vi "Initiate and Generate (Multi).vi"(0 "niUsrpRio Sessions":T3[](array[typedef]) {"FPGA Data Clock Rate" format="%#.3pHz"; "Data Clock Rate" format="%#.3pHz"; "Characterization Data"."Frequencies [Hz]" format="%#_6p"; "EEPROM Characterization Header"."Pointer to Device Data Header" format="%x"; "EEPROM Characterization Header"."Checksum" format="%x"; "Device Data Header"."Pointer to Characterization Data" format="%x"; "Device Data Header"."Checksum" format="%x"; "EEPROM Header"."Pointer to User Header" format="%x"; "EEPROM Header"."Pointer to Factory Header" format="%x"; "EEPROM Header"."Product Code" format="%x"; "EEPROM Header"."Checksum" format="%x"}, 1 "tx channels":T2(array[cluster]) {"tx.coerced configurations"."coerced sample rates" format="%#.3pS/s"; "tx.coerced configurations"."coerced levels" format="%#.3gdBm"; "tx.coerced configurations"."coerced lo frequencies" format="%#.3pHz"; "tx.coerced configurations"."coerced frequencies" format="%#.3pHz"; "tx config"."tone frequency" format="%#.3pHz"; "tx config"."sample rate" format="%#.3pS/s"; "tx config"."rf config 0"."level" format="%#_gdBm"; "tx config"."rf config 0"."lo frequency" format="%#.3pHz"; "tx config"."rf config 0"."frequency" format="%#.3pHz"; "tx config"."rf config 1"."level" format="%#_gdBm"; "tx config"."rf config 1"."lo frequency" format="%#.3pHz"; "tx config"."rf config 1"."frequency" format="%#.3pHz"}, 5 "start trigger time":dbl=1.0 format="%#.6ps", 7 "update interval":dbl=0.1 format="%#.6ps", 9 "first iteration":bool, 11 "error in":errorcluster) -> (4 "niUsrpRio Sessions (out)":T3[](array[typedef]) {"FPGA Data Clock Rate" format="%#.3pHz"; "Data Clock Rate" format="%#.3pHz"; "Characterization Data"."Frequencies [Hz]" format="%#_6p"; "EEPROM Characterization Header"."Pointer to Device Data Header" format="%x"; "EEPROM Characterization Header"."Checksum" format="%x"; "Device Data Header"."Pointer to Characterization Data" format="%x"; "Device Data Header"."Checksum" format="%x"; "EEPROM Header"."Pointer to User Header" format="%x"; "EEPROM Header"."Pointer to Factory Header" format="%x"; "EEPROM Header"."Product Code" format="%x"; "EEPROM Header"."Checksum" format="%x"}, 15 "error out":errorcluster)   [LabVIEW 2015]
uses:
  <instrlib>/niUsrpRio/Config/v1/Host/Public/niUsrpRio Session.ctl
  <instrlib>/_niInstr/Register Bus/v0/Host/Public/Register Bus Session.ctl
  <instrlib>/_niInstr/Register Bus/v0/Host/Private/Session Data.ctl
  <instrlib>/niUsrpRio/Config/v1/Host/Private/DB Queue Reference.ctl
  <instrlib>/niUsrpRio/Config/v1/Host/Private/Daughterboard Data.ctl
  <instrlib>/niUsrpRio/Config/v1/Host/Private/ATR state data.ctl
  <instrlib>/niUsrpRio/Config/v1/Host/Public/EEPROM Header.ctl
  <instrlib>/niUsrpRio/Config/v1/Host/Public/EEPROM Device Data Header.ctl
  <instrlib>/niUsrpRio/Config/v1/Host/Public/EEPROM Characterization Header.ctl
  <instrlib>/niUsrpRio/Config/v1/Host/Public/Characterization Data.ctl
  <instrlib>/niUsrpRio/Config/v1/Host/Public/IQ Imbalance.ctl
  Start Trigger.ctl
  Write Tx Data (I16 multi).vi
  <instrlib>/_niInstr/Register Bus/v0/Host/niInstr Register Bus v0 Host.lvlib
  <instrlib>/niUsrpRio/Config/v1/Host/niUsrpRio Config v1 Host.lvlib
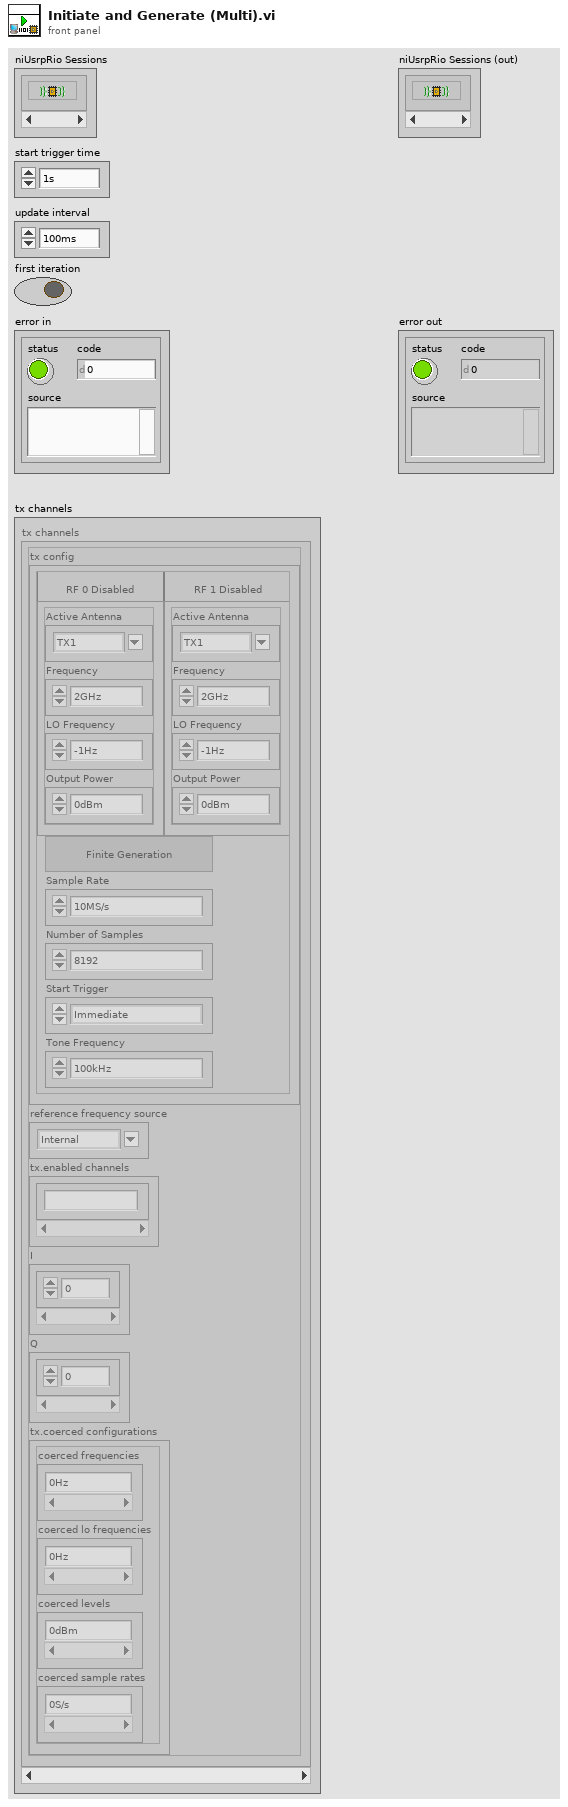
[diagram p1: front panel]
types:
  T1 = typedef "Start Trigger.ctl" = enum8{"Software", "Digital Edge", "Rx Start Trigger", "Tx Start Trigger", "Immediate", "Future Time Event"}
  T2 = cluster{"tx config":cluster{"rf enable 0":bool, "rf config 0":cluster{"antenna":string, "frequency":dbl, "lo frequency":dbl, "level":dbl}, "rf enable 1":bool, "rf config 1":cluster{"antenna":string, "frequency":dbl, "lo frequency":dbl, "level":dbl}, "number of samples is finite":bool, "sample rate":dbl, "number of samples":u32, "start trigger":T1, "tone frequency":dbl}, "reference frequency source":string, "tx.enabled channels":string[], "I":i16[], "Q":i16[], "tx.coerced configurations":cluster{"coerced frequencies":dbl[], "coerced lo frequencies":dbl[], "coerced levels":dbl[], "coerced sample rates":dbl[]}}[]
  T3 = typedef "niUsrpRio Config v1 Host.lvlib/niUsrpRio Session.ctl" = cluster{"FPGA Interface":refnum<k20>, "RIO Interface Number":u32, "Data Clock Rate":u32, "FPGA Data Clock Rate":u32, "Global Settings Register Bus":T4, "Radio 0 Settings Register Bus":T4, "Radio 1 Settings Register Bus":T4, "Radio Settings Bus Semaphore":T5, "DB Queues":T6[], "Characterization Data Valid?":bool, "EEPROM Header":T7, "Device Data Header":T8, "EEPROM Characterization Header":T9, "Characterization Data":T10[], "FPGA Current Version":u32, "FPGA Oldest Compatible Version":u32, "Fixed Logic Current Version":u32, "Fixed Logic Oldest Compatible Version":u32, "FPGA Radio Settings Bus Current Version":u32, "FPGA Radio Settings Bus Oldest Compatible Version":u32, "FPGA Board Config Current Version":u32, "FPGA Board Config Oldest Compatible Version":u32}
  T4 = typedef "niInstr Register Bus v0 Host.lvlib/Register Bus Session.ctl" = refnum<queue>
  T5 = typedef "Semaphore RefNum" = refnum<k1>
  T6 = typedef "niUsrpRio Config v1 Host.lvlib/DB Queue Reference.ctl" = refnum<queue>
  T7 = typedef "niUsrpRio Config v1 Host.lvlib/EEPROM Header.ctl" = cluster{"Checksum":u32, "Product Code":u16, "Hardware Current Version":u16, "Hardware Oldest Compatible Version":u16, "EEPROM Map Current Version":u16, "EEPROM Map Oldest Compatible Version":u16, "User Password":string, "Pointer to Factory Header":u32, "Pointer to User Header":u32, "Recommended Interval":u16, "Number of Reserved Bytes":i32, "Number of Daughterboards":u8, "Daughterboard IDs":u16[], "Daughterboard Serial Numbers":string[]}
  T8 = typedef "niUsrpRio Config v1 Host.lvlib/EEPROM Device Data Header.ctl" = cluster{"Checksum":u32, "Number of Channels":u8, "Number of Gain Settings":u16[], "Pointer to Characterization Data":u32[], "Number of Reserved Bytes":i32, "Number of Frequencies":u16[]}
  T9 = typedef "niUsrpRio Config v1 Host.lvlib/EEPROM Characterization Header.ctl" = cluster{"Checksum":u32, "Date":timestamp, "Temperature":sgl, "Misc. Info":string, "Pointer to Device Data Header":u32, "Number of Reserved Bytes":i32}
  T10 = typedef "niUsrpRio Config v1 Host.lvlib/Characterization Data.ctl" = cluster{"Gains[dB]":dbl[], "Frequencies [Hz]":dbl[], "IQ Imbalance Table":T11[], "Measured Gains[dB]":dbl[][]}
  T11 = typedef "niUsrpRio Config v1 Host.lvlib/IQ Imbalance.ctl" = cluster{"Gain Imbalance [linear]":dbl, "Phase Imbalance [radians]":dbl, "Offset":cdb}
  T12 = cluster{"tx config":cluster{"rf enable 0":bool, "rf config 0":cluster{"antenna":string, "frequency":dbl, "lo frequency":dbl, "level":dbl}, "rf enable 1":bool, "rf config 1":cluster{"antenna":string, "frequency":dbl, "lo frequency":dbl, "level":dbl}, "number of samples is finite":bool, "sample rate":dbl, "number of samples":u32, "start trigger":T1, "tone frequency":dbl}, "reference frequency source":string, "tx.enabled channels":string[], "I":i16[], "Q":i16[], "tx.coerced configurations":cluster{"coerced frequencies":dbl[], "coerced lo frequencies":dbl[], "coerced levels":dbl[], "coerced sample rates":dbl[]}}
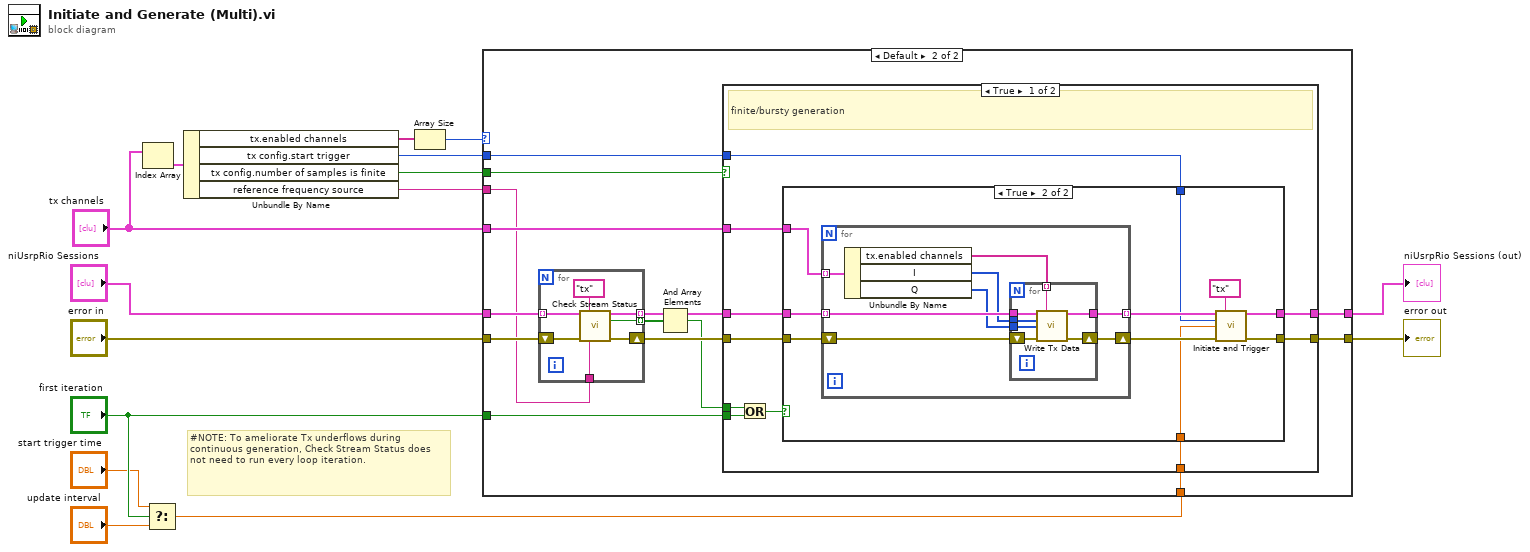
[diagram p0: block diagram]
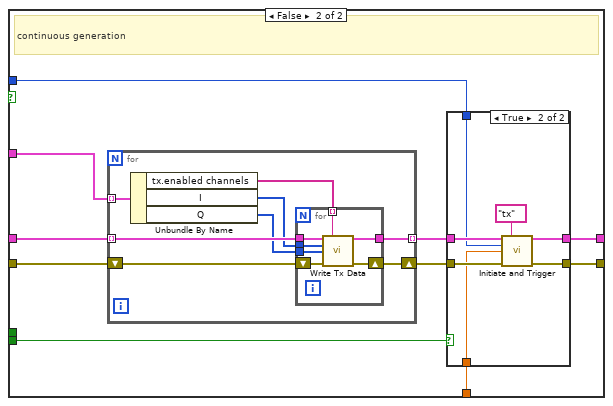
[diagram p4: hidden frame]
diagram:
  # "#NOTE: To ameliorate Tx underflows during continuous generation, Check Stream Status does not need to run every loop iteration."
  n1 = Index Array(array="tx channels") -> (element=w10:T12)  [unwired: 1 in]
  n2 = Select(t="start trigger time", s="first iteration", f="update interval") -> (s? t:f=w1:dbl)
  n3 = Unbundle By Name(w10) -> ("tx.enabled channels"=w6:string[], "tx config.start trigger"=w7:T1, "tx config.number of samples is finite"=w11:bool, "reference frequency source"=w8:string)
  n4 = Array Size(array=w6) -> (size(s)=w5:i32)
  n5 = case shown="Default" w5 {
    tunnel: "niUsrpRio Sessions" -> [w16 w30]
    tunnel: "error in" -> [w17 w29]
    tunnel: [w16 w26] -> w13
    tunnel: [w17 w25] -> w12
    tunnel: "first iteration" -> [_ w19]
    tunnel: w11 -> [_ w24]
    tunnel: "tx channels" -> [_ w23]
    tunnel: w8 -> [_ w22]
    tunnel: w7 -> [_ w21]
    tunnel: w1 -> [_ w18]
    frame 0 {
      # "do nothing if there are zero enabled channels"
    }
    frame Default {
      n6 = for {
        tunnel: [w38] -> w31 mode=indexing
        shift-right: [w37] -> w27
        shift-left: w29 -> [w36]
        tunnel: w30 -> [w35] mode=indexing
        tunnel: [w34] -> w28 mode=indexing
        tunnel: w22 -> [w32]
        n7 = call "Check Stream Status.vi"("niUsrpRio Session"=w35, "scope"="tx", "error in"=w36, "reference frequency source"=w32) -> ("niUsrpRio Session (out)"=w34:T3, "done"=w38:bool, "error out"=w37:errorcluster)  [unwired: 9 in]
      }
      n8 = And Array Elements(Boolean array=w31) -> (logical AND=w20:bool)
      n9 = case shown="True" w24 {
        tunnel: w28 -> [w48 w85]
        tunnel: w27 -> [w47 w84]
        tunnel: [w46 w83] -> w26
        tunnel: [w45 w82] -> w25
        tunnel: w23 -> [w44 w81]
        tunnel: w21 -> [w43 w80]
        tunnel: w19 -> [w42 w77]
        tunnel: w20 -> [w41 _]
        tunnel: w18 -> [w39 w76]
        frame True {
          # "finite/bursty generation"
          n10 = Or(x=w41, y=w42) -> (x .or. y?=w40:bool)
          n11 = case shown="True" w40 {
            tunnel: w48 -> [w49 w60]
            tunnel: w47 -> [w50 w59]
            tunnel: [w49 w55] -> w46
            tunnel: [w50 w56] -> w45
            tunnel: w44 -> [_ w57]
            tunnel: w43 -> [_ w52]
            tunnel: w39 -> [_ w51]
            frame False {
              # "Do nothing until the previous finite generation finishes before reinitiating."
            }
            frame True {
              n12 = for {
                tunnel: [w65] -> w54 mode=indexing
                tunnel: w60 -> [w67] mode=indexing
                shift-right: [w66] -> w58
                shift-left: w59 -> [w68]
                tunnel: w57 -> [w63] mode=indexing
                n13 = Unbundle By Name(w63) -> ("tx.enabled channels"=w64:string[], "I"=w62:i16[], "Q"=w61:i16[])
                n14 = for {
                  shift-right: [w74] -> w66
                  shift-left: w68 -> [w75]
                  tunnel: w67 -> [w73]
                  tunnel: [w72] -> w65
                  tunnel: w64 -> [w71] mode=indexing
                  tunnel: w62 -> [w70]
                  tunnel: w61 -> [w69]
                  n15 = call-poly "Write Tx Data.vi"("niUsrpRio Session"=w73, "scope"=w71, "I"=w70, "Q"=w69, "error in"=w75) -> ("niUsrpRio Session (out)"=w72:T3, "error out"=w74:errorcluster)  [unwired: 9 in]
                }
              }
              n16 = call "Initiate and Trigger.vi"("niUsrpRio Sessions"=w54, "scope"="tx", "start trigger"=w52, "trigger delay"=w51, "error in"=w58) -> ("niUsrpRio Sessions (out)"=w55:T3[], "error out"=w56:errorcluster)  [unwired: 9 in]
            }
          }
        }
        frame False {
          # "continuous generation"
          n17 = for {
            tunnel: [w99] -> w78 mode=indexing
            tunnel: w85 -> [w101] mode=indexing
            shift-right: [w100] -> w79
            shift-left: w84 -> [w102]
            tunnel: w81 -> [w97] mode=indexing
            n18 = Unbundle By Name(w97) -> ("tx.enabled channels"=w98:string[], "I"=w96:i16[], "Q"=w95:i16[])
            n19 = for {
              shift-right: [w108] -> w100
              shift-left: w102 -> [w109]
              tunnel: w101 -> [w107]
              tunnel: [w106] -> w99
              tunnel: w98 -> [w105] mode=indexing
              tunnel: w96 -> [w104]
              tunnel: w95 -> [w103]
              n20 = call-poly "Write Tx Data.vi"("niUsrpRio Session"=w107, "scope"=w105, "I"=w104, "Q"=w103, "error in"=w109) -> ("niUsrpRio Session (out)"=w106:T3, "error out"=w108:errorcluster)  [unwired: 9 in]
            }
          }
          n21 = case shown="True" w77 {
            tunnel: [w87 w93] -> w83
            tunnel: [w86 w92] -> w82
            tunnel: w80 -> [_ w91]
            tunnel: w79 -> [w86 w90]
            tunnel: w78 -> [w87 w94]
            tunnel: w76 -> [_ w88]
            frame False {
              # "Only initiate on first iteration."
            }
            frame True {
              n22 = call "Initiate and Trigger.vi"("niUsrpRio Sessions"=w94, "scope"="tx", "start trigger"=w91, "trigger delay"=w88, "error in"=w90) -> ("niUsrpRio Sessions (out)"=w93:T3[], "error out"=w92:errorcluster)  [unwired: 9 in]
            }
          }
        }
      }
    }
  }
  "niUsrpRio Sessions (out)" <- w13
  "error out" <- w12
